vi "Shoot Switch.vi"(1 "Shoot Switch Long":bool, 2 "Shoot Switch Short":bool, 3 "error in (no error)":errorcluster) -> (10 "error out":errorcluster)   [LabVIEW 2017]
uses:
  <vilib>/Rock Robotics/WPI/Utilities/WPI_GetSetVariantRefNum.vi
  <vilib>/Rock Robotics/WPI/ThirdParty/Phoenix-LabVIEW/Motor Controller/Controls/CTRE_Phoenix_MotorControl_ControlMode.ctl
panel:
  # "Short: shoot -0.15\nLong: shoot -0.3"
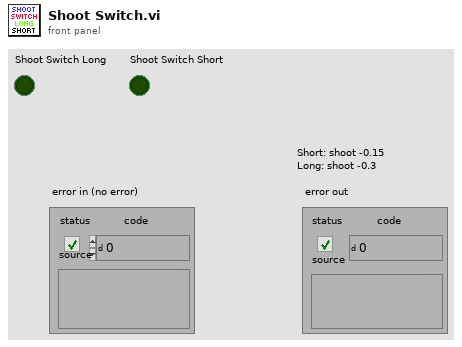
[diagram p1: front panel]
types:
  T1 = typedef "WPI_RobotDriveDevRef.ctl" = cluster{"DevStatus":errorcluster, "Motors[]":T2[], "Square Inputs":bool, "Max Output":dbl}
  T2 = typedef "WPI_MotorControlDeviceRef.ctl" = cluster{"DeviceStatus":errorcluster, "Type":T3, "PWM":cluster{"PWM Channel":T4, "DeadBand":T5}, "CAN":cluster{"Device Number":u8, "SetOutput VI Ref":variant, "GetOutput VI Ref":variant, "Enable VI Ref":variant, "Disable VI Ref":variant, "Data":variant}, "Invert":bool, "DIO PWM":cluster{"PWM \"Enable\" Channel":T4, "DIOChannel":T6, "PWM Rate":dbl}}
  T3 = typedef "WPI_MotorControlType.ctl" = enum16{"PWM", "CAN", "DIO PWM"}
  T4 = typedef "FPGA_DIOPWMChannel.ctl" = enum8{"PWM 0", "PWM 1", "PWM 2", "PWM 3", "PWM 4", "PWM 5", "PWM 6", "PWM 7", "PWM 8", "PWM 9", "PWM MXP 0", "PWM MXP 1", "PWM MXP 2", "PWM MXP 3", "PWM MXP 4", "PWM MXP 5", "PWM MXP 6", "PWM MXP 7", "PWM MXP 8", "PWM MXP 9", "Invalid"}
  T5 = typedef "WPI_PWMDeadband.ctl" = cluster{"Name":string, "maxPositivePwm":i32, "minPositivePwm":i32, "centerPwm":i32, "maxNegativePwm":i32, "minNegativePwm":i32, "angularRange":u16}
  T6 = typedef "FPGA_DIOChannel.ctl" = enum8{"DIO 0", "DIO 1", "DIO 2", "DIO 3", "DIO 4", "DIO 5", "DIO 6", "DIO 7", "DIO 8", "DIO 9", "DIO MXP 0", "DIO MXP 1", "DIO MXP 2", "DIO MXP 3", "DIO MXP 4", "DIO MXP 5", "DIO MXP 6", "DIO MXP 7", "DIO MXP 8", "DIO MXP 9", "DIO MXP 10", "DIO MXP 11", "DIO MXP 12", "DIO MXP 13", "DIO MXP 14", "DIO MXP 15", "SPI Port CS1", "SPI Port CS2", "SPI Port CS3", "SPI Port MISO", "SPI Port MOSI", "Invalid"}
  T7 = typedef "CTRE_Phoenix_MotorControl_ControlMode.ctl" = u16
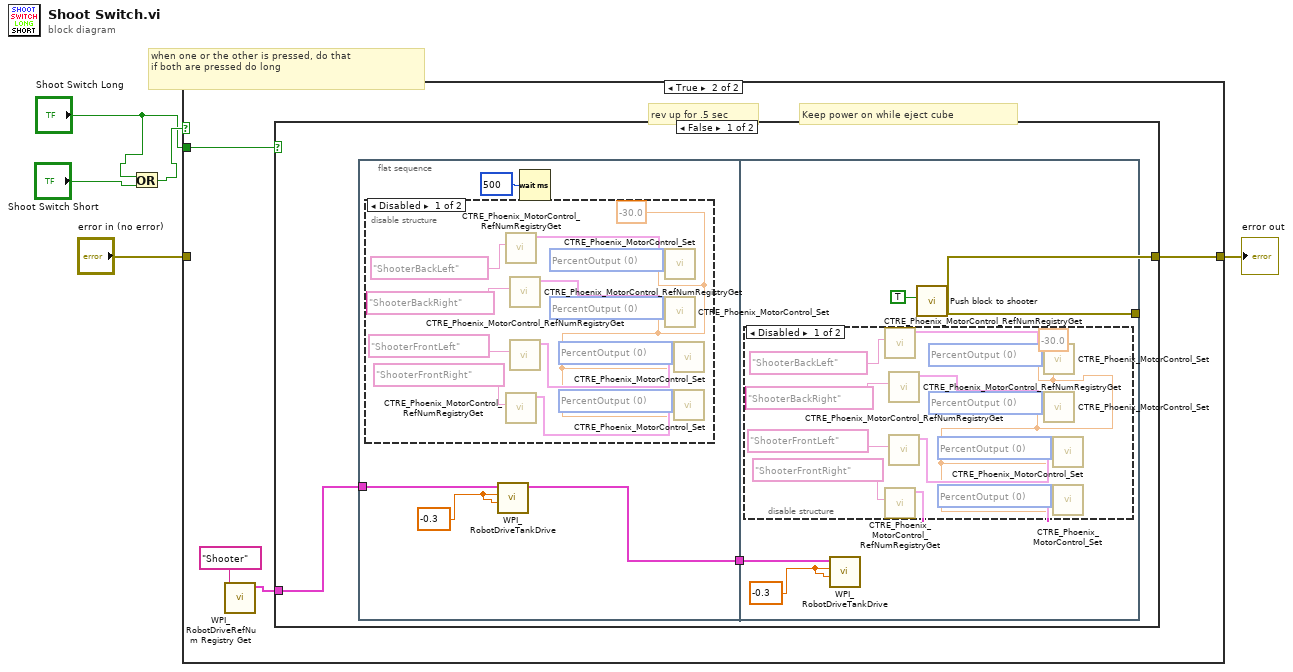
[diagram p0: block diagram]
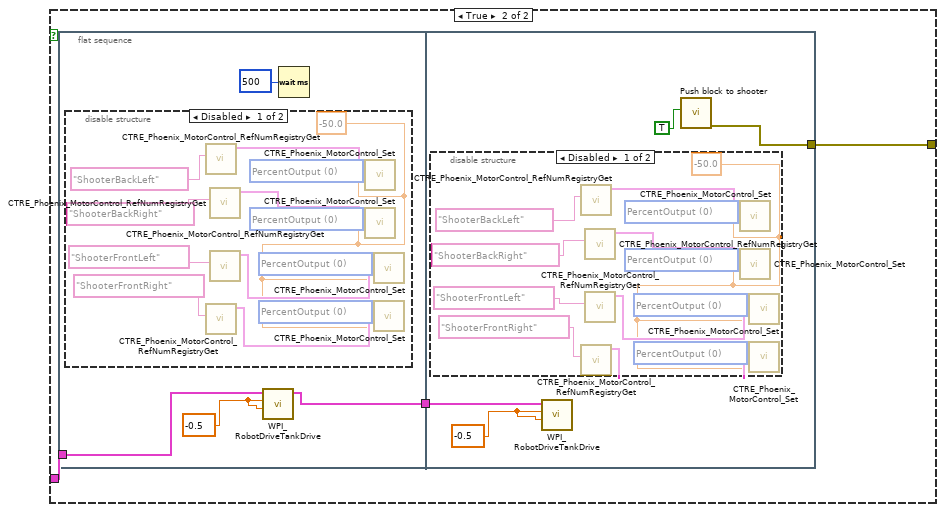
[diagram p5: hidden frame]
diagram:
  # "when one or the other is pressed, do that\nif both are pressed do long"
  n1 = Or(x="Shoot Switch Long", y="Shoot Switch Short") -> (x .or. y?=w3:bool)
  n2 = case shown="True" w3 {
    tunnel: "Shoot Switch Long" -> [_ w10]
    tunnel: "error in (no error)" -> [w6 _]
    tunnel: [w6 w9] -> w4
    frame False {
    }
    frame True {
      # "Keep power on while eject cube"
      # "rev up for .5 sec"
      n3 = call <vilib>:"WPI_RobotDriveRefNum Registry Get.vi"("refnum name"="Shooter") -> ("RobotDriveDevRef"=w7:T1)  [unwired: 9 in, 1 out]
      n4 = case shown="False" w10 {
        tunnel: [w13 w50] -> w9
        tunnel: w7 -> [w12 w49]
        frame False {
          n5 = flat-sequence {
            tunnel: w12 -> [w15]
            tunnel: [w14] -> w11
            tunnel: [w33] -> w13
            tunnel: w11 -> [w31]
            frame #0 {
              w16 = -0.3
              n6 = disable-structure shown="Disabled" {
                frame Disabled {
                  w18 = -30.0
                  w26 = T7 0 items=["PercentOutput"=0, "Position"=1, "Velocity"=2, "Current"=3, "Follower"=5, "MotionProfile"=6, "MotionMagic"=7, "MotionMagicArc"=8, "MotionProfileArc"=10, "Disabled"=15] ("Control Mode")
                  w25 = T7 0 items=["PercentOutput"=0, "Position"=1, "Velocity"=2, "Current"=3, "Follower"=5, "MotionProfile"=6, "MotionMagic"=7, "MotionMagicArc"=8, "MotionProfileArc"=10, "Disabled"=15] ("Control Mode")
                  w24 = T7 0 items=["PercentOutput"=0, "Position"=1, "Velocity"=2, "Current"=3, "Follower"=5, "MotionProfile"=6, "MotionMagic"=7, "MotionMagicArc"=8, "MotionProfileArc"=10, "Disabled"=15] ("Control Mode")
                  w23 = T7 0 items=["PercentOutput"=0, "Position"=1, "Velocity"=2, "Current"=3, "Follower"=5, "MotionProfile"=6, "MotionMagic"=7, "MotionMagicArc"=8, "MotionProfileArc"=10, "Disabled"=15] ("Control Mode")
                  n7 = call <vilib>:"CTRE_Phoenix_MotorControl_RefNumRegistryGet.vi"("refnum name"="ShooterBackLeft") -> ("PhoenixMotorControlDevRef"=w22:T2)  [unwired: 9 in, 1 out]
                  n8 = call <vilib>:"CTRE_Phoenix_MotorControl_RefNumRegistryGet.vi"("refnum name"="ShooterFrontRight") -> ("PhoenixMotorControlDevRef"=w19:T2)  [unwired: 9 in, 1 out]
                  n9 = call <vilib>:"CTRE_Phoenix_MotorControl_RefNumRegistryGet.vi"("refnum name"="ShooterBackRight") -> ("PhoenixMotorControlDevRef"=w21:T2)  [unwired: 9 in, 1 out]
                  n10 = call <vilib>:"CTRE_Phoenix_MotorControl_RefNumRegistryGet.vi"("refnum name"="ShooterFrontLeft") -> ("PhoenixMotorControlDevRef"=w20:T2)  [unwired: 9 in, 1 out]
                  n11 = call <vilib>:"CTRE_Phoenix_MotorControl_Set.vi"("Output"=w18, "Control Mode"=w23, "PhoenixMotorControlDevRef"=w22) -> ()  [unwired: 7 in, 2 out]
                  n12 = call <vilib>:"CTRE_Phoenix_MotorControl_Set.vi"("Output"=w18, "Control Mode"=w24, "PhoenixMotorControlDevRef"=w21) -> ()  [unwired: 7 in, 2 out]
                  n13 = call <vilib>:"CTRE_Phoenix_MotorControl_Set.vi"("Output"=w18, "Control Mode"=w25, "PhoenixMotorControlDevRef"=w20) -> ()  [unwired: 7 in, 2 out]
                  n14 = call <vilib>:"CTRE_Phoenix_MotorControl_Set.vi"("Output"=w18, "Control Mode"=w26, "PhoenixMotorControlDevRef"=w19) -> ()  [unwired: 7 in, 2 out]
                }
                frame Enabled {
                }
              }
              n15 = call <vilib>:"WPI_RobotDriveTankDrive.vi"("Right axis value"=w16, "Left axis value"=w16, "RobotDriveDevRef"=w15) -> ("RobotDriveDevRef"=w14:T1)  [unwired: 6 in, 2 out]
              n16 = Wait (ms)(milliseconds to wait=u32 500) -> ()  [unwired: 1 out]
            }
            frame #1 {
              w32 = -0.3
              n17 = disable-structure shown="Disabled" {
                frame Disabled {
                  w35 = -30.0
                  w40 = T7 0 items=["PercentOutput"=0, "Position"=1, "Velocity"=2, "Current"=3, "Follower"=5, "MotionProfile"=6, "MotionMagic"=7, "MotionMagicArc"=8, "MotionProfileArc"=10, "Disabled"=15] ("Control Mode")
                  w41 = T7 0 items=["PercentOutput"=0, "Position"=1, "Velocity"=2, "Current"=3, "Follower"=5, "MotionProfile"=6, "MotionMagic"=7, "MotionMagicArc"=8, "MotionProfileArc"=10, "Disabled"=15] ("Control Mode")
                  w42 = T7 0 items=["PercentOutput"=0, "Position"=1, "Velocity"=2, "Current"=3, "Follower"=5, "MotionProfile"=6, "MotionMagic"=7, "MotionMagicArc"=8, "MotionProfileArc"=10, "Disabled"=15] ("Control Mode")
                  w43 = T7 0 items=["PercentOutput"=0, "Position"=1, "Velocity"=2, "Current"=3, "Follower"=5, "MotionProfile"=6, "MotionMagic"=7, "MotionMagicArc"=8, "MotionProfileArc"=10, "Disabled"=15] ("Control Mode")
                  n18 = call <vilib>:"CTRE_Phoenix_MotorControl_RefNumRegistryGet.vi"("refnum name"="ShooterBackLeft") -> ("PhoenixMotorControlDevRef"=w44:T2)  [unwired: 9 in, 1 out]
                  n19 = call <vilib>:"CTRE_Phoenix_MotorControl_RefNumRegistryGet.vi"("refnum name"="ShooterFrontRight") -> ("PhoenixMotorControlDevRef"=w47:T2)  [unwired: 9 in, 1 out]
                  n20 = call <vilib>:"CTRE_Phoenix_MotorControl_RefNumRegistryGet.vi"("refnum name"="ShooterBackRight") -> ("PhoenixMotorControlDevRef"=w45:T2)  [unwired: 9 in, 1 out]
                  n21 = call <vilib>:"CTRE_Phoenix_MotorControl_RefNumRegistryGet.vi"("refnum name"="ShooterFrontLeft") -> ("PhoenixMotorControlDevRef"=w46:T2)  [unwired: 9 in, 1 out]
                  n22 = call <vilib>:"CTRE_Phoenix_MotorControl_Set.vi"("Output"=w35, "Control Mode"=w43, "PhoenixMotorControlDevRef"=w44) -> ()  [unwired: 7 in, 2 out]
                  n23 = call <vilib>:"CTRE_Phoenix_MotorControl_Set.vi"("Output"=w35, "Control Mode"=w42, "PhoenixMotorControlDevRef"=w45) -> ()  [unwired: 7 in, 2 out]
                  n24 = call <vilib>:"CTRE_Phoenix_MotorControl_Set.vi"("Output"=w35, "Control Mode"=w41, "PhoenixMotorControlDevRef"=w46) -> ()  [unwired: 7 in, 2 out]
                  n25 = call <vilib>:"CTRE_Phoenix_MotorControl_Set.vi"("Output"=w35, "Control Mode"=w40, "PhoenixMotorControlDevRef"=w47) -> ()  [unwired: 7 in, 2 out]
                }
                frame Enabled {
                }
              }
              n26 = call <vilib>:"WPI_RobotDriveTankDrive.vi"("Right axis value"=w32, "Left axis value"=w32, "RobotDriveDevRef"=w31) -> ()  [unwired: 6 in, 3 out]
              n27 = call "Push block to shooter.vi"("Shoot?"=TRUE) -> ("error out"=w33:errorcluster)  [unwired: 10 in]
            }
          }
        }
        frame True {
          n28 = flat-sequence {
            tunnel: w49 -> [w53]
            tunnel: [w51] -> w48
            tunnel: [w70] -> w50
            tunnel: w48 -> [w68]
            frame #0 {
              w52 = -0.5
              n29 = disable-structure shown="Disabled" {
                frame Disabled {
                  w55 = -50.0
                  w63 = T7 0 items=["PercentOutput"=0, "Position"=1, "Velocity"=2, "Current"=3, "Follower"=5, "MotionProfile"=6, "MotionMagic"=7, "MotionMagicArc"=8, "MotionProfileArc"=10, "Disabled"=15] ("Control Mode")
                  w62 = T7 0 items=["PercentOutput"=0, "Position"=1, "Velocity"=2, "Current"=3, "Follower"=5, "MotionProfile"=6, "MotionMagic"=7, "MotionMagicArc"=8, "MotionProfileArc"=10, "Disabled"=15] ("Control Mode")
                  w61 = T7 0 items=["PercentOutput"=0, "Position"=1, "Velocity"=2, "Current"=3, "Follower"=5, "MotionProfile"=6, "MotionMagic"=7, "MotionMagicArc"=8, "MotionProfileArc"=10, "Disabled"=15] ("Control Mode")
                  w60 = T7 0 items=["PercentOutput"=0, "Position"=1, "Velocity"=2, "Current"=3, "Follower"=5, "MotionProfile"=6, "MotionMagic"=7, "MotionMagicArc"=8, "MotionProfileArc"=10, "Disabled"=15] ("Control Mode")
                  n30 = call <vilib>:"CTRE_Phoenix_MotorControl_RefNumRegistryGet.vi"("refnum name"="ShooterBackLeft") -> ("PhoenixMotorControlDevRef"=w59:T2)  [unwired: 9 in, 1 out]
                  n31 = call <vilib>:"CTRE_Phoenix_MotorControl_RefNumRegistryGet.vi"("refnum name"="ShooterFrontRight") -> ("PhoenixMotorControlDevRef"=w56:T2)  [unwired: 9 in, 1 out]
                  n32 = call <vilib>:"CTRE_Phoenix_MotorControl_RefNumRegistryGet.vi"("refnum name"="ShooterBackRight") -> ("PhoenixMotorControlDevRef"=w58:T2)  [unwired: 9 in, 1 out]
                  n33 = call <vilib>:"CTRE_Phoenix_MotorControl_RefNumRegistryGet.vi"("refnum name"="ShooterFrontLeft") -> ("PhoenixMotorControlDevRef"=w57:T2)  [unwired: 9 in, 1 out]
                  n34 = call <vilib>:"CTRE_Phoenix_MotorControl_Set.vi"("Output"=w55, "Control Mode"=w60, "PhoenixMotorControlDevRef"=w59) -> ()  [unwired: 7 in, 2 out]
                  n35 = call <vilib>:"CTRE_Phoenix_MotorControl_Set.vi"("Output"=w55, "Control Mode"=w61, "PhoenixMotorControlDevRef"=w58) -> ()  [unwired: 7 in, 2 out]
                  n36 = call <vilib>:"CTRE_Phoenix_MotorControl_Set.vi"("Output"=w55, "Control Mode"=w62, "PhoenixMotorControlDevRef"=w57) -> ()  [unwired: 7 in, 2 out]
                  n37 = call <vilib>:"CTRE_Phoenix_MotorControl_Set.vi"("Output"=w55, "Control Mode"=w63, "PhoenixMotorControlDevRef"=w56) -> ()  [unwired: 7 in, 2 out]
                }
                frame Enabled {
                }
              }
              n38 = call <vilib>:"WPI_RobotDriveTankDrive.vi"("Right axis value"=w52, "Left axis value"=w52, "RobotDriveDevRef"=w53) -> ("RobotDriveDevRef"=w51:T1)  [unwired: 6 in, 2 out]
              n39 = Wait (ms)(milliseconds to wait=u32 500) -> ()  [unwired: 1 out]
            }
            frame #1 {
              w69 = -0.5
              n40 = disable-structure shown="Disabled" {
                frame Disabled {
                  w72 = -50.0
                  w80 = T7 0 items=["PercentOutput"=0, "Position"=1, "Velocity"=2, "Current"=3, "Follower"=5, "MotionProfile"=6, "MotionMagic"=7, "MotionMagicArc"=8, "MotionProfileArc"=10, "Disabled"=15] ("Control Mode")
                  w79 = T7 0 items=["PercentOutput"=0, "Position"=1, "Velocity"=2, "Current"=3, "Follower"=5, "MotionProfile"=6, "MotionMagic"=7, "MotionMagicArc"=8, "MotionProfileArc"=10, "Disabled"=15] ("Control Mode")
                  w78 = T7 0 items=["PercentOutput"=0, "Position"=1, "Velocity"=2, "Current"=3, "Follower"=5, "MotionProfile"=6, "MotionMagic"=7, "MotionMagicArc"=8, "MotionProfileArc"=10, "Disabled"=15] ("Control Mode")
                  w77 = T7 0 items=["PercentOutput"=0, "Position"=1, "Velocity"=2, "Current"=3, "Follower"=5, "MotionProfile"=6, "MotionMagic"=7, "MotionMagicArc"=8, "MotionProfileArc"=10, "Disabled"=15] ("Control Mode")
                  n41 = call <vilib>:"CTRE_Phoenix_MotorControl_RefNumRegistryGet.vi"("refnum name"="ShooterBackLeft") -> ("PhoenixMotorControlDevRef"=w76:T2)  [unwired: 9 in, 1 out]
                  n42 = call <vilib>:"CTRE_Phoenix_MotorControl_RefNumRegistryGet.vi"("refnum name"="ShooterFrontRight") -> ("PhoenixMotorControlDevRef"=w73:T2)  [unwired: 9 in, 1 out]
                  n43 = call <vilib>:"CTRE_Phoenix_MotorControl_RefNumRegistryGet.vi"("refnum name"="ShooterBackRight") -> ("PhoenixMotorControlDevRef"=w75:T2)  [unwired: 9 in, 1 out]
                  n44 = call <vilib>:"CTRE_Phoenix_MotorControl_RefNumRegistryGet.vi"("refnum name"="ShooterFrontLeft") -> ("PhoenixMotorControlDevRef"=w74:T2)  [unwired: 9 in, 1 out]
                  n45 = call <vilib>:"CTRE_Phoenix_MotorControl_Set.vi"("Output"=w72, "Control Mode"=w77, "PhoenixMotorControlDevRef"=w76) -> ()  [unwired: 7 in, 2 out]
                  n46 = call <vilib>:"CTRE_Phoenix_MotorControl_Set.vi"("Output"=w72, "Control Mode"=w78, "PhoenixMotorControlDevRef"=w75) -> ()  [unwired: 7 in, 2 out]
                  n47 = call <vilib>:"CTRE_Phoenix_MotorControl_Set.vi"("Output"=w72, "Control Mode"=w79, "PhoenixMotorControlDevRef"=w74) -> ()  [unwired: 7 in, 2 out]
                  n48 = call <vilib>:"CTRE_Phoenix_MotorControl_Set.vi"("Output"=w72, "Control Mode"=w80, "PhoenixMotorControlDevRef"=w73) -> ()  [unwired: 7 in, 2 out]
                }
                frame Enabled {
                }
              }
              n49 = call <vilib>:"WPI_RobotDriveTankDrive.vi"("Right axis value"=w69, "Left axis value"=w69, "RobotDriveDevRef"=w68) -> ()  [unwired: 6 in, 3 out]
              n50 = call "Push block to shooter.vi"("Shoot?"=TRUE) -> ("error out"=w70:errorcluster)  [unwired: 10 in]
            }
          }
        }
      }
    }
  }
  "error out" <- w4
